vi "Load Settings from XML.vi"(8 "error in (no error)":cluster{"状态":bool, "代码":i32, "源":string} caption="错误输入（无错误）", 11 "设置输入":T1) -> (0 "error out":cluster{"状态":bool, "代码":i32, "源":string} caption="错误输出", 3 "设置输出":T1)   [LabVIEW 2012, in "Settings.lvlib"]
doc: "尝试从XML文件加载先前的用户设置。\n\n该VI不会生成错误。如无法加载和解析XML文件，直接返回默认设置。"
uses:
  Settings.lvlib
  Settings.ctl
  Acquisition/Hardware Configuration.ctl
  Acquisition/Signal Type.ctl
  Logging/Logging Configuration.ctl
  <vilib>/Utility/xml.llb/Read From XML File(string).vi
  <vilib>/Utility/xml.llb/Write to XML File(string).vi
  Acquisition/Acquisition.lvlib
  Logging/Logging.lvlib
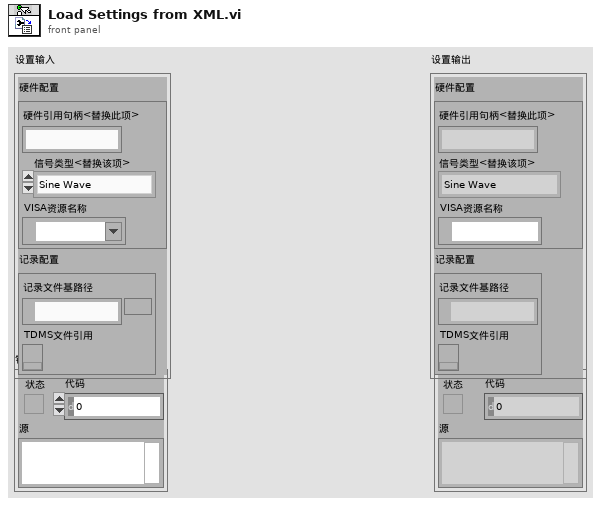
[diagram p1: front panel]
types:
  T1 = typedef "Settings.lvlib/Settings.ctl" = cluster{"硬件配置":T2, "记录配置":T4}
  T2 = typedef "Acquisition.lvlib/Hardware Configuration.ctl" = cluster{"硬件引用句柄<替换此项>":string, "信号类型<替换该项>":T3, "VISA资源名称":refnum<visa-resource-name>}
  T3 = typedef "Acquisition.lvlib/Signal Type.ctl" = enum16{"Sine Wave", "Square with Noise"}
  T4 = typedef "Logging.lvlib/Logging Configuration.ctl" = cluster{"记录文件基路径":path, "TDMS文件引用":refnum<k34>}
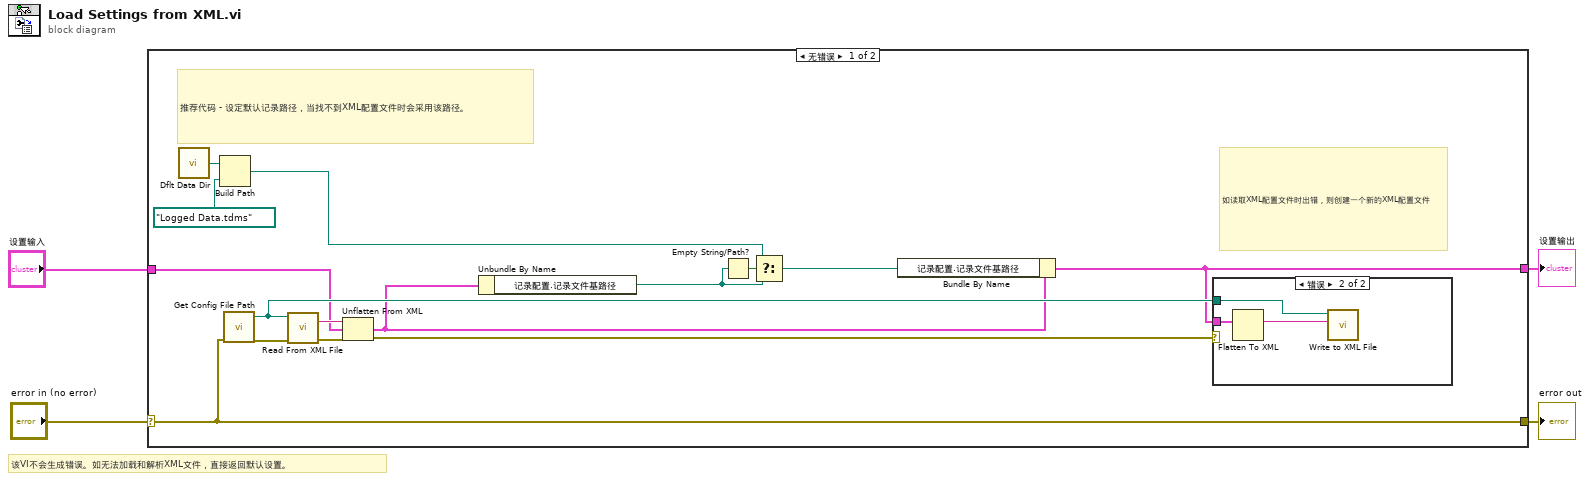
[diagram p0: block diagram]
diagram:
  # "该VI不会生成错误。如无法加载和解析XML文件，直接返回默认设置。"
  n1 = case shown="无错误" "error in (no error)" {
    selector: "error in (no error)" -> [w17 w24]
    tunnel: [w17 w24] -> w3
    tunnel: "设置输入" -> [w11 w23]
    tunnel: [w5 w23] -> w1
    frame No Error {
      # "如读取XML配置文件时出错，则创建一个新的XML配置文件"
      # "推荐代码 - 设定默认记录路径，当找不到XML配置文件时会采用该路径。"
      n2 = call <vilib>:"Dflt Data Dir.vi"() -> ("App:Default Data Directory"=w16:path)
      n3 = Build Path(base path=w16, name or relative path=path "Logged Data.tdms" ("App:Default Data Directory")) -> (appended path=w8:path)
      n4 = call "Get Config File Path.vi"("error in (no error)"=w17) -> ("error out"=w19:cluster{"状态":bool, "代码":i32, "源":string}, "XML文件路径"=w14:path)  [unwired: 9 in]
      n5 = call-poly <vilib>:"Read From XML File.vi"("error in (no error)"=w19, "XML File Path"=w14) -> ("error out"=w13:errorcluster, "XML Elements"=w18:string)  [unwired: 7 in, 1 out]
      n6 = Unflatten From XML(xml string=w18, type=w11, error in (no error)=w13) -> (value=w7:T1, error out=w12:errorcluster)
      n7 = Unbundle By Name(w7) -> ("记录配置.记录文件基路径"=w9:path)
      n8 = Empty String/Path?(string/path=w9) -> (empty?=w10:bool)
      n9 = Select(t=w8, s=w10, f=w9) -> (s? t:f=w6:path)
      n10 = Bundle By Name(cluster=w7, "记录配置.记录文件基路径"=w6) -> (w5:T1)
      n11 = case shown="错误" w12 {
        tunnel: w5 -> [_ w22]
        tunnel: w14 -> [_ w20]
        frame No Error {
        }
        frame Error {
          n12 = Flatten To XML(anything=w22) -> (xml string=w21:string)
          n13 = call-poly <vilib>:"Write to XML File.vi"("XML Input"=w21, "XML File Path"=w20) -> ()  [unwired: 7 in, 3 out]
        }
      }
    }
    frame Error {
    }
  }
  "error out" <- w3
  "设置输出" <- w1
